vi "Assert Not In Range.vi"(3 "Execution time (s)":dbl=-1.0, 4 "Register with caller test (F)":bool, 5 "Assert Only? (F)":bool, 6 "error code (1)":i32=1, 7 "Label (\"\")":string, 8 "error in (no error)":errorcluster, 9 "Lower Limit":ext, 10 "Upper Limit":ext, 11 "X":ext) -> (0 "error out":errorcluster, 2 "Properties.Assert":refnum<class "Properties.Assert.lvclass">)   [LabVIEW 2013, in "Caraya.lvlib" / "Assert.lvclass"]
doc: "Asserts that <B>X</B> is not between <B>upper limit</B> and <B>lower limit</B>."
uses:
  Assert.lvclass
  Properties.Assert/Properties.Assert.lvclass
  Properties/Properties.lvclass
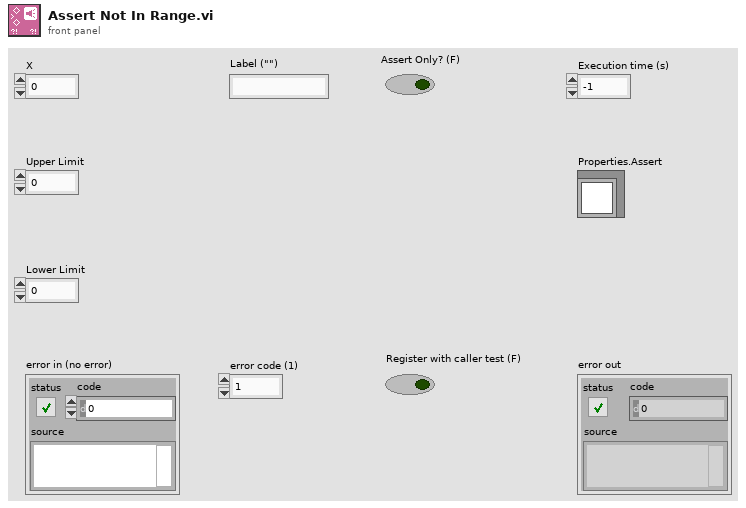
[diagram p1: front panel]
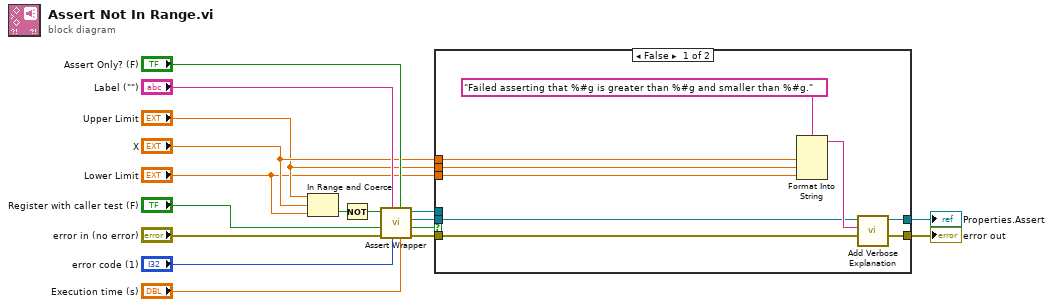
[diagram p0: block diagram]
diagram:
  n1 = In Range and Coerce(upper limit="Upper Limit", x="X", lower limit="Lower Limit") -> (In Range?=w5:bool)  [unwired: 1 out]
  n2 = Not(x=w5) -> (.not. x?=w1:bool)
  n3 = call "Assert Wrapper.vi"("Execution time (s)"="Execution time (s)", "Assert Only? (F)"="Assert Only? (F)", "error code (1)"="error code (1)", "Label"="Label (\"\")", "error in (no error)"="error in (no error)", "Register with caller test (F)"="Register with caller test (F)", "Assert?"=w1) -> ("error out"=w8:errorcluster, "Verbose"=w12:bool, "Properties.Assert"=w10:refnum<class "Properties.Assert.lvclass">, "Assert out"=w11:refnum<class "Assert.lvclass">)  [unwired: 1 in]
  n4 = case shown="False" w12 {
    tunnel: w11 -> [_ _]
    tunnel: w10 -> [w23 w28]
    tunnel: [w25 w27] -> w9
    tunnel: w8 -> [w26 w27]
    tunnel: [w22 w28] -> w7
    tunnel: "X" -> [w20 _]
    tunnel: "Upper Limit" -> [w19 _]
    tunnel: "Lower Limit" -> [w18 _]
    frame False {
      n5 = Format Into String(format string="Failed asserting that %#g is greater than %#g and smaller than %#g.", w20, w19, w18) -> (resulting string=w24:string)  [unwired: 2 in, 1 out]
      n6 = call "Add Verbose Explanation.vi"("error in (no error)"=w26, "Verbose Explanation"=w24, "Properties"=w23) -> ("error out"=w25:errorcluster, "Properties"=w22:refnum<class "Properties.Assert.lvclass">)  [unwired: 7 in]
    }
    frame True {
    }
  }
  "error out" <- w9
  "Properties.Assert" <- w7
